vi "Display One Button Popup (Plain).vi"(4 "keep transparent buttons?":bool=TRUE, 6 "Theme":refnum<class "Theme.lvclass">, 7 "Button Text":string="OK", 8 "error in":errorcluster, 10 "Message":string, 11 "Dialog Title":string) -> (0 "error out":errorcluster)   [LabVIEW 2021, in "Pop-Up.lvlib" / "Plain - One Button.lvclass"]
doc: "The one button popup will display information to the user and wait for the operator to click the button.\n\n<b>Note:</b> The function <b>Close Pop-Up.vi</b> can be used to close this dialog early.\n\n<b>Note:</b> The dialog vertical sizing will adjust for longer messages, so <b>test</b> all messages prior to deployment to make sure that scaling fits.\n\nInputs: +\n-Dialog Title [String] - String variable to populate the dialog's title bar +\n-Message [String] - String variable to populate Display +\n-Theme [lvclass] - the theme for the style of the popup +\n-Button Text [String] - String variable for defining the text to show on the button +\n-Keep transparent buttons? [Boolean] - choose to leave buttons transparent (T) or use theme colors (F)\n\n<b>Code Developed By:</b> +\nDaniel Coons +\nhttps://github.com/danielcoons/tsc-pop-up"
uses:
  Plain - One Button.lvclass
  Theme/Theme.lvclass
  C:/Development/Open Source/tsc-pop-up/Popup/Popup.lvclass
  C:/Development/Open Source/tsc-pop-up/Plain/Plain Parent.lvclass
  Plain Parent.lvclass/Plain Parent.ctl
  Write Dialog Title.vi
  Write Action 1 Text.vi
  Set Transparent buttons.vi
  Popup/Data Member Access/Write Theme.vi
  Plain - One Button.lvclass/Plain - One Button.ctl
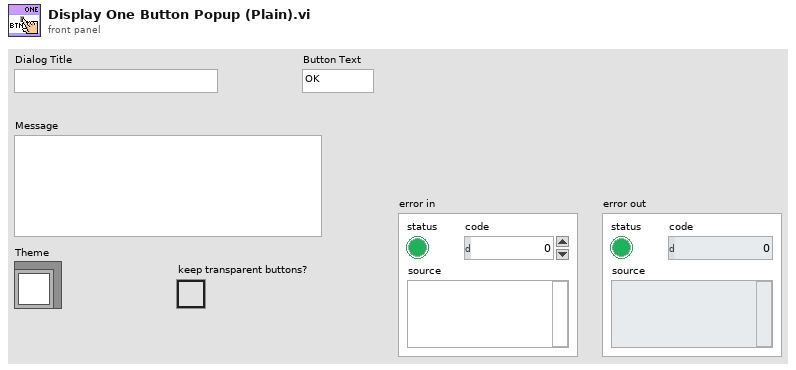
[diagram p1: front panel]
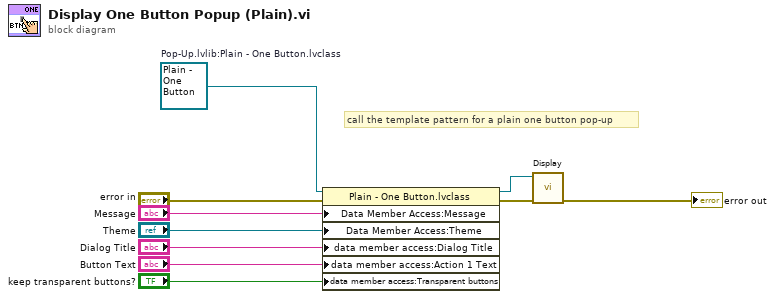
[diagram p0: block diagram]
diagram:
  w2 = refnum<class "Plain - One Button.lvclass"> refnum  # Pop-Up.lvlib:Plain - One Button.lvclass
  # "call the template pattern for a plain one button pop-up"
  n1 = property class="Plain - One Button.lvclass"(reference=w2, error in="error in", "Data Member Access:Message"="Message", "Data Member Access:Theme"="Theme", "data member access:Dialog Title"="Dialog Title", "data member access:Action 1 Text"="Button Text", "data member access:Transparent buttons"="keep transparent buttons?") -> (reference out=w7:refnum<class "Plain - One Button.lvclass">, error out=w8:errorcluster)
  n2 = call-dynamic "Display.vi"("error in"=w8, "Plain - One Button in"=w7) -> ("error out"=→"error out":errorcluster)  [unwired: 8 in, 1 out]
